vi "Begin.vi"(11 "Image Size":T1=enum."160x120") -> (0 "error out":errorcluster)   [LabVIEW 2011]
doc: "Called before other user functions, this VI is expected to open initial I/O refnums, load in file data, and do all program initialization. Notice that the <B>error out</B> terminal is simply used for data flow. Wiring it to other structures or subVIs ensures that this VI runs first."
uses:
  <vilib>/Rock Robotics/WPI/Camera/WPI_CameraImageSize.ctl
  <vilib>/Rock Robotics/WPI/Joystick/WPI_JoystickDeviceEnum.ctl
  <vilib>/Rock Robotics/WPI/CAN/Jaguar/SubVIs/WPI_CANJaguar_ControlMode.ctl
  <vilib>/Rock Robotics/WPI/MotorControl/WPI_MotorControlOpenCANJaguar.vi
  <vilib>/Rock Robotics/WPI/Camera/WPI_CameraWhite Balance Values.ctl
  <vilib>/Rock Robotics/WPI/Camera/WPI_CameraExposure Values.ctl
  <vilib>/Rock Robotics/WPI/Camera/WPI_CameraFrameRate.ctl
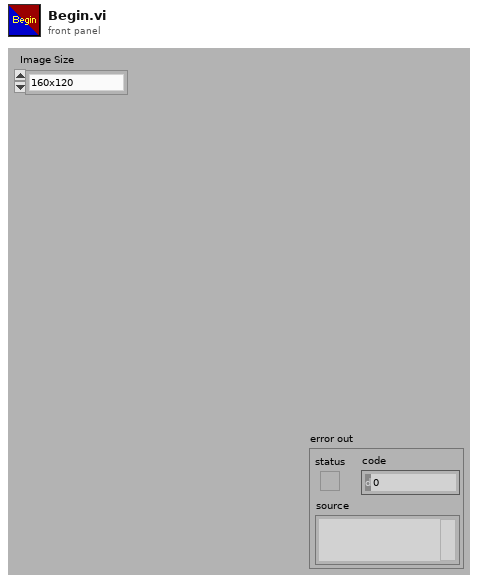
[diagram p1: front panel]
types:
  T1 = typedef "WPI_CameraImageSize.ctl" = enum16{"640x480", "320x240", "160x120"}
  T2 = typedef "WPI_CANJaguar_ControlMode.ctl" = enum8{"Percent VBus", "Current", "Speed", "Position", "Voltage"}
  T3 = typedef "WPI_JoystickDeviceEnum.ctl" = enum16{"USB 1", "USB 2", "USB 3", "USB 4", "Kinect 1", "Kinect 2"}
  T4 = typedef "WPI_CameraFrameRate.ctl" = u32
  T5 = typedef "WPI_CameraExposure Values.ctl" = enum16{"Auto", "Flicker-free 50 Hz", "Flicker-free 60 Hz", "Hold current"}
  T6 = typedef "WPI_CameraWhite Balance Values.ctl" = enum16{"Auto", "Fixed indoor", "Fixed outdoor 1", "Fixed outdoor 2", "Fixed fluorescent 1", "Fixed fluorescent 2", "Hold current"}
  T7 = typedef "WPI_CameraDevRef.ctl" = cluster{"Camera Address":string, "CameraStatus":errorcluster, "Acquire Image Notifier":refnum<notifier>}
  T8 = typedef "WPI_MotorControlDeviceRef.ctl" = cluster{"DeviceStatus":errorcluster, "Type":enum16{"PWM", "CAN"}, "PWM":cluster{"Digital Module":T9, "PWM Channel":T10, "DeadBand":T11}, "CAN":cluster{"Device Number":u8, "Control Mode":T2, "Semaphore":T12, "Max Vout":dbl}, "Invert":bool, "TransformRef":T13, "InvTransformRef":T13}
  T9 = typedef "FPGA_TypedefDigitalModule.ctl" = enum16{"Digital Module 1", "Digital Module 2"}
  T10 = typedef "FPGA_DIOPWMChannel.ctl" = enum8{"PWM 1", "PWM 2", "PWM 3", "PWM 4", "PWM 5", "PWM 6", "PWM 7", "PWM 8", "PWM 9", "PWM 10", "Invalid"}
  T11 = typedef "WPI_PWMDeadband.ctl" = cluster{"Name":string, "maxPositivePwm":i32, "minPositivePwm":i32, "centerPwm":i32, "maxNegativePwm":i32, "minNegativePwm":i32, "angularRange":u16}
  T12 = typedef "Semaphore RefNum" = refnum<k1>
  T13 = typedef "WPI_PWMTransform_ConPane.ctl" = refnum<vi>
  T14 = typedef "WPI_JoystickDevRef.ctl" = cluster{"Device":T3}
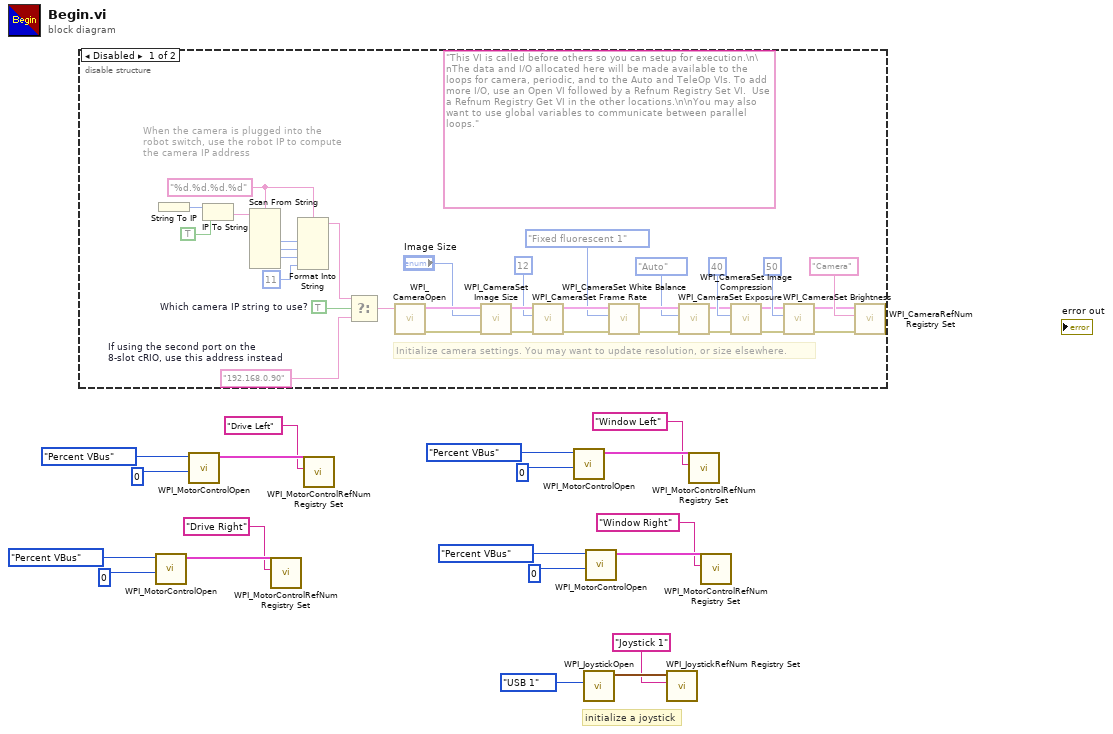
[diagram p0: block diagram]
diagram:
  # "initialize a joystick"
  n1 = disable-structure shown="Disabled" {
    frame Disabled {
      w20 = TRUE  # Which camera IP string to use?
      w24 = "%d.%d.%d.%d" ("format string")
      (unwired) "This VI is called before others so you can setup for execution.\n\nThe data and I/O allocated here will be made available to the loops for camera, periodic, and to the Auto and TeleOp VIs. To add more I/O, use an Open VI followed by a Refnum Registry Set VI.  Use a Refnum Registry Get VI in the other locations.\n\nYou may also want to use global variables to communicate between parallel loops."
      w21 = "192.168.0.90"  # If using the second port on the 8-slot cRIO, use this address instead
      # "When the camera is plugged into the\nrobot switch, use the robot IP to compute\nthe camera IP address"
      # "Initialize camera settings. You may want to update resolution, or size elsewhere."
      n2 = String To IP() -> (0:w31:u32)  [unwired: 1 in]
      n3 = IP To String(1:TRUE ("dot notation? (F)"), 2:w31) -> (0:w29:string)
      n4 = Scan From String(format string=w24, input string=w29) -> (output 1=w28:i32, output 2=w27:i32, output 3=w26:i32)  [unwired: 7 in, 3 out]
      n5 = Format Into String(format string=w24, w28, w27, w26, 11 ("Compression")) -> (resulting string=w22:string)  [unwired: 2 in, 1 out]
      n6 = Select(t=w22, s=w20, f=w21) -> (s? t:f=w23:string)
      n7 = call <vilib>:"WPI_CameraOpen.vi"("Camera Address"=w23) -> ("error out"=w43:errorcluster, "CameraDevRef"=w44:T7)  [unwired: 1 in, 8 out]
      n8 = call <vilib>:"WPI_CameraSet Image Size.vi"("error in (no error)"=w43, "Image Size"="Image Size", "CameraDevRef"=w44) -> ("error out"=w42:errorcluster, "CameraDevRef Out"=w45:T7)  [unwired: 7 out]
      n9 = call <vilib>:"WPI_CameraSet Frame Rate.vi"("error in (no error)"=w42, "Frame Rate (fps)"=T4 12, "CameraDevRef"=w45) -> ("error out"=w41:errorcluster, "CameraDevRef Out"=w47:T7)  [unwired: 7 out]
      n10 = call <vilib>:"WPI_CameraSet White Balance.vi"("error in (no error)"=w41, "White Balance"=WPI_CameraWhite_Balance_Values."Fixed fluorescent 1", "CameraDevRef"=w47) -> ("error out"=w40:errorcluster, "CameraDevRef Out"=w46:T7)  [unwired: 7 out]
      n11 = call <vilib>:"WPI_CameraSet Exposure.vi"("error in (no error)"=w40, "Exposure"=WPI_CameraExposure_Values."Auto", "CameraDevRef"=w46) -> ("error out"=w39:errorcluster, "CameraDevRef Out"=w49:T7)  [unwired: 7 out]
      n12 = call <vilib>:"WPI_CameraSet Image Compression.vi"("error in (no error)"=w39, "Compression"=40, "CameraDevRef"=w49) -> ("error out"=w38:errorcluster, "CameraDevRef Out"=w48:T7)  [unwired: 7 out]
      n13 = call <vilib>:"WPI_CameraSet Brightness.vi"("error in (no error)"=w38, "Brightness"=50, "CameraDevRef"=w48) -> ("error out"=w36:errorcluster, "CameraDevRef Out"=w37:T7)  [unwired: 7 out]
      n14 = call <vilib>:"WPI_CameraRefNum Registry Set.vi"("error in (no error)"=w36, "refnum name"="Camera", "CameraDevRef"=w37) -> ()  [unwired: 9 out]
    }
    frame Enabled {
    }
  }
  n15 = call-poly <vilib>:"WPI_MotorControlOpen.vi"("Device Number"=u8 0, "Control Mode"=WPI_CANJaguar_ControlMode."Percent VBus") -> ("MotorControlDeviceRef"=w2:T8)  [unwired: 8 in, 1 out]
  n16 = call-poly <vilib>:"WPI_MotorControlOpen.vi"("Device Number"=u8 0, "Control Mode"=WPI_CANJaguar_ControlMode."Percent VBus") -> ("MotorControlDeviceRef"=w6:T8)  [unwired: 8 in, 1 out]
  n17 = call <vilib>:"WPI_MotorControlRefNum Registry Set.vi"("refnum name"="Drive Right", "MotorControlDevRef"=w2) -> ()  [unwired: 8 in, 2 out]
  n18 = call <vilib>:"WPI_MotorControlRefNum Registry Set.vi"("refnum name"="Drive Left", "MotorControlDevRef"=w6) -> ()  [unwired: 8 in, 2 out]
  n19 = call-poly <vilib>:"WPI_MotorControlOpen.vi"("Device Number"=u8 0, "Control Mode"=WPI_CANJaguar_ControlMode."Percent VBus") -> ("MotorControlDeviceRef"=w14:T8)  [unwired: 8 in, 1 out]
  n20 = call <vilib>:"WPI_JoystickOpen.vi"("JoystickDevice"=WPI_JoystickDeviceEnum."USB 1") -> ("JoystickDevRef"=w19:T14)  [unwired: 10 out]
  n21 = call-poly <vilib>:"WPI_MotorControlOpen.vi"("Device Number"=u8 0, "Control Mode"=WPI_CANJaguar_ControlMode."Percent VBus") -> ("MotorControlDeviceRef"=w10:T8)  [unwired: 8 in, 1 out]
  n22 = call <vilib>:"WPI_JoystickRefNum Registry Set.vi"("refnum name"="Joystick 1", "JoystickDevRef"=w19) -> ()  [unwired: 1 in, 9 out]
  n23 = call <vilib>:"WPI_MotorControlRefNum Registry Set.vi"("refnum name"="Window Left", "MotorControlDevRef"=w14) -> ()  [unwired: 8 in, 2 out]
  n24 = call <vilib>:"WPI_MotorControlRefNum Registry Set.vi"("refnum name"="Window Right", "MotorControlDevRef"=w10) -> ()  [unwired: 8 in, 2 out]
